vi "Interpolate.vi"   [LabVIEW 2016, in "xy_utilities.lvlib"]
doc: "Use this VI to interpolate data and add \"fake\" points outside of the given x array.\n\nWire data to the data input to determine the polymorphic instance to use or manually select the instance."
uses:
  xy_utilities.lvlib
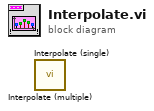
[diagram p0: block diagram]
diagram:
  n1 = call "Interpolate (multiple).vi"() -> ()  [unwired: 10 in, 2 out]
  n2 = call "Interpolate (single).vi"() -> ()  [unwired: 10 in, 2 out]
